vi "signal_analysis.vi"() -> ()   [LabVIEW 2012]
uses:
  <vilib>/measure/mascope.llb/Amplitude and Levels 1 chan.vi
  <vilib>/express/express analysis/Spectral/Block/exnSpectralBlock spectral measurements RMS poly.vi
  <vilib>/express/express analysis/Spectral/Block/exnSpectralBlock spectral measurements RMS DDT.vi
  <vilib>/express/express analysis/Spectral/XNode/ExpressSpectralMeasurementsBlockNode.xnode
  <vilib>/measure/NI_MAPro.lvlib
panel:
  out "Peak-Peak amplitude (V)":dbl format="%.2p"
  out "Amplitude (V)":dbl format="%#_3g"
  out "Filtered Signal":dynamicdata(graph)
  in  "Frequency":dbl(knob)=10.1 scale=1.0..100.0
  out "FFT":dynamicdata(graph)
  in  "stop":bool
  in  "Amplitude":dbl=1.0
  out "Sine":dynamicdata(graph)
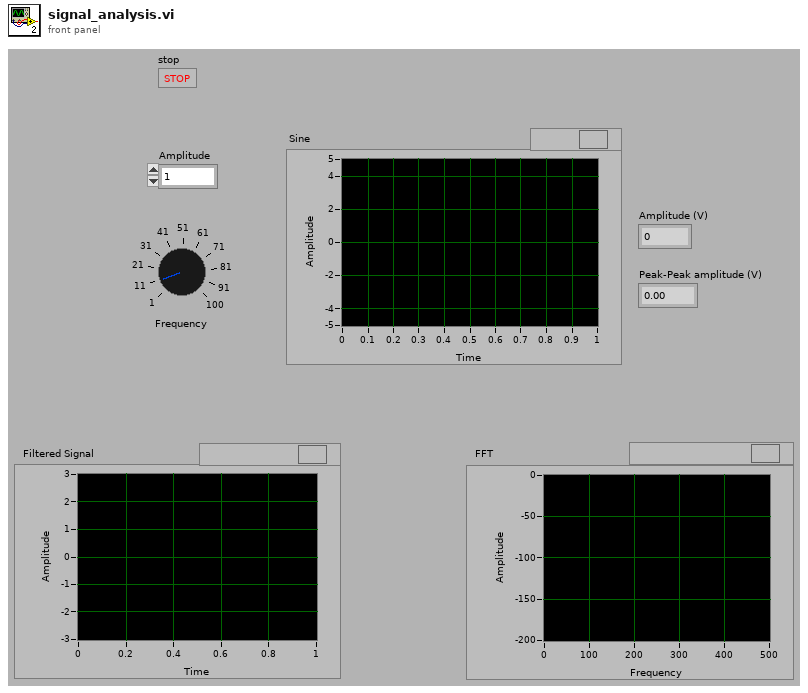
[diagram p1: front panel]
types:
  T1 = cluster{"averaging mode":u16, "weighting mode":u16, "number of averages":u32}
  T2 = cluster{"dB On (F)":bool, "unwrap phase (F)":bool, "convert to degree (F)":bool}
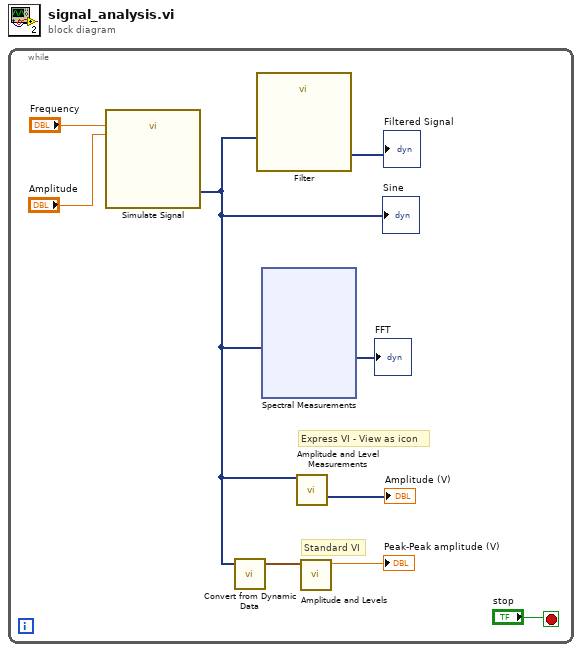
[diagram p0: block diagram]
diagram:
  n1 = while {
    stop <- "stop" stop-if-true
    # "Standard VI"
    # "Express VI - View as icon"
    n2 = call "Simulate Signal"("Frequency"="Frequency", "Amplitude"="Amplitude") -> ("Sine"=w3:dynamicdata)  [unwired: 12 in, 1 out]
    "Sine" <- w3
    n3 = call "Convert from Dynamic Data"("Dynamic Data Type"=w3) -> ("Waveform"=w2:waveform(dbl))  [unwired: 3 in]
    n4 = call "Filter"("Signal"=w3) -> ("Filtered Signal"=→"Filtered Signal":dynamicdata)  [unwired: 9 in, 1 out]
    n5 = xnode "Spectral Measurements"("Signals"=w3) -> ("FFT - (RMS)"=→"FFT":dynamicdata)  [unwired: 1 in, 2 out]
    n6 = call "Amplitude and Level Measurements"("Signals"=w3) -> ("Positive Peak"=→"Amplitude (V)":dynamicdata)  [unwired: 13 in, 1 out]
    n7 = call-poly <vilib>:"Amplitude and Levels.vi"("signal in"=w2) -> ("amplitude"=→"Peak-Peak amplitude (V)":dbl)  [unwired: 7 in, 3 out]
  }
